vi "UTILITY Modbus 32bit Number to 16bit Array.vi"(8 "error in":errorcluster, 11 "32-bit IEEE 754":sgl) -> (0 "error out":errorcluster, 3 "U16 Array Representation":u16[](array[numeric]) format="%x")   [LabVIEW 2020]
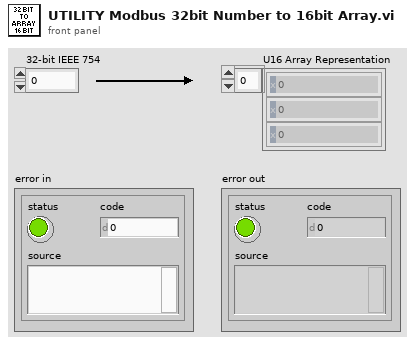
[diagram p1: front panel]
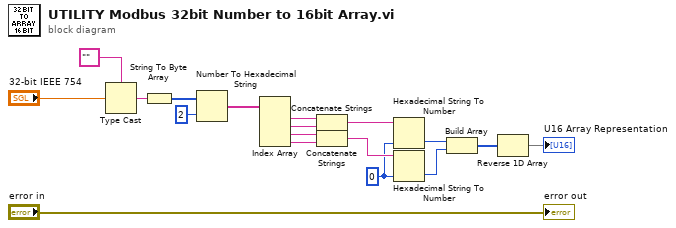
[diagram p0: block diagram]
diagram:
  w6 = u16 0 ("default (0 U32)")
  n1 = Type Cast(type="", x="32-bit IEEE 754") -> (*(type *) &x=w16:string)
  n2 = String To Byte Array(string=w16) -> (unsigned byte array=w15:u8[])
  n3 = Number To Hexadecimal String(1:i16 2 ("width (-)"), 2:w15) -> (0:w13:string[])
  n4 = Index Array(array=w13) -> (element #1=w12:string, element #2=w11:string, element #3=w10:string, element #4=w9:string)  [unwired: 4 in]
  n5 = Concatenate Strings(w12, w11) -> (w8:string)
  n6 = Concatenate Strings(w10, w9) -> (w7:string)
  n7 = Hexadecimal String To Number(string=w8, default (0uL)=w6) -> (number=w5:u16)  [unwired: 1 in, 1 out]
  n8 = Hexadecimal String To Number(string=w7, default (0uL)=w6) -> (number=w4:u16)  [unwired: 1 in, 1 out]
  n9 = Build Array(w5, w4) -> (w2:u16[])
  n10 = Reverse 1D Array(array=w2) -> (reversed array=→"U16 Array Representation":u16[])
  "error out" <- "error in"
